vi "Material-DefectDetection.vi"(0 "Conditioned output":dbl[](array[numeric]), 1 "Subtraction to Apply":bool) -> (5 "Flagged for Defect":bool, 6 "Array":dbl[](array[numeric]))   [LabVIEW 2013, in "Material-RunTest.lvclass"]
uses:
  Material-RunTest.lvclass
  <userlib>/_OpenG.lib/array/array.llb/Search 1D Array (Boolean)__ogtk.vi
  <userlib>/_OpenG.lib/array/array.llb/Empty 1D Array (I32)__ogtk.vi
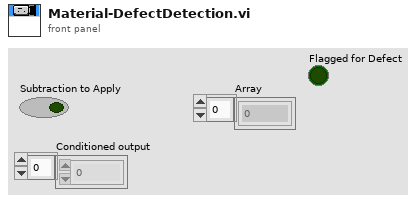
[diagram p1: front panel]
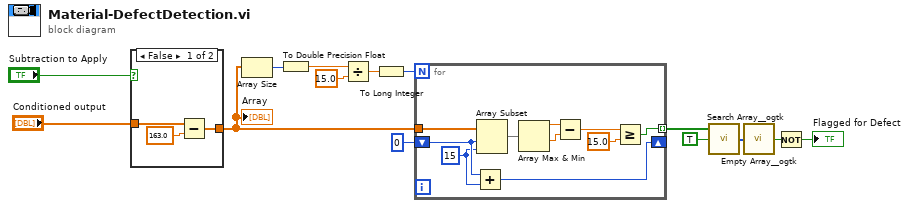
[diagram p0: block diagram]
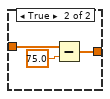
[diagram p2: hidden frame]
diagram:
  n1 = case shown="False" "Subtraction to Apply" {
    tunnel: "Conditioned output" -> [w16 w20]
    tunnel: [w15 w18] -> w7
    frame False {
      n2 = Subtract(x=w16, y=163.0) -> (x-y=w15:dbl[])
    }
    frame True {
      n3 = Subtract(x=w20, y=75.0) -> (x-y=w18:dbl[])
    }
  }
  "Array" <- w7
  n4 = Array Size(array=w7) -> (size(s)=w11:i32)
  n5 = To Double Precision Float(number=w11) -> (double precision float=w12:dbl)
  n6 = Divide(x=w12, y=15.0) -> (x/y=w9:dbl)
  n7 = To Long Integer(number=w9) -> (32bit integer=w8:i32)
  n8 = for {
    N: w8 -> [_]
    tunnel: w7 -> [w30]
    shift-right: [w27] -> _
    shift-left: 0 -> [w29]
    tunnel: [w21] -> w5 mode=indexing
    w28 = 15 ("length")
    n9 = Add(x=w29, y=w28) -> (x+y=w27:i32)
    n10 = Array Subset(array=w30, index=w29, length=w28) -> (w26:dbl[])
    n11 = Array Max & Min(array=w26) -> (max value=w25:dbl, min value=w24:dbl)  [unwired: 2 out]
    n12 = Subtract(x=w25, y=w24) -> (x-y=w23:dbl)
    n13 = Greater Or Equal?(x=w23, y=15.0) -> (x >= y?=w21:bool)
  }
  n14 = call-poly <userlib>:"Search Array__ogtk.vi"("Array"=w5, "Element Data"=TRUE) -> ("Indices of Elements"=w3:i32[])  [unwired: 7 in]
  n15 = call-poly <userlib>:"Empty Array__ogtk.vi"("Array"=w3) -> ("Empty Array?"=w2:bool)  [unwired: 8 in]
  n16 = Not(x=w2) -> (.not. x?=→"Flagged for Defect":bool)
